vi "UDC Archive And Upload.vi"(8 "Error In":errorcluster) -> (0 "Error Out":errorcluster)   [LabVIEW 2017, in "niceiplib.lvlib"]
doc: "UDC_SYMBOLS void UDCArchiveAndUpload();\n\nThis VI initiates the archive and upload of the data collected in the files."
uses:
  <vilib>/UDC/niceiplib.lvlib
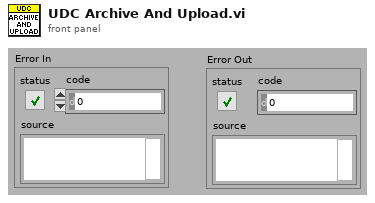
[diagram p1: front panel]
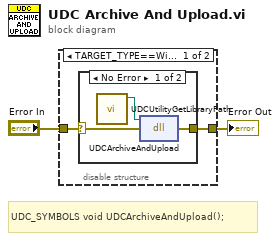
[diagram p0: block diagram]
diagram:
  # "UDC_SYMBOLS void UDCArchiveAndUpload();"
  n1 = disable-structure shown="TARGET_TYPE==Windows" {
    disable-tunnel: "Error In" -> [w4 w9]
    disable-tunnel: [w3 w9] -> w1
    frame condition #0 (active) {
      n2 = case shown="No Error" w4 {
        selector: w4 -> [w7 w8]
        tunnel: [w6 w8] -> w3
        frame No Error {
          n3 = call <vilib>:"UDCUtilityGetLibraryPath.vi"() -> ("Library Path"=w5:path)  [unwired: 11 in]
          n4 = dll-call lib="C:/2013LabVIEWCode/dist/vi.lib/UDC/niceiplib.*" fn="UDCArchiveAndUpload"(path in=w5, error in=w7) -> (error out=w6:errorcluster)  [unwired: 2 in, 1 out]
        }
        frame Error {
        }
      }
    }
    frame condition #1 {
    }
  }
  "Error Out" <- w1
